vi "SV TDMS Read Position Info.vi"(0 "tdms file":refnum<k34>, 5 "group name in":string, 7 "channel name in":string, 11 "error in":errorcluster) -> (4 "tdms file out":refnum<k34>, 6 "group name out":string, 8 "channel name out":string, 10 "position info":T1, 15 "error out":errorcluster)   [LabVIEW 2017]
uses:
  <vilib>/addons/_NISVFA/_Shared subVIs/Controls/svc_Position Info.ctl
  <vilib>/addons/_NISVFA/_Shared subVIs/Controls/SV Channel Properties.ctl
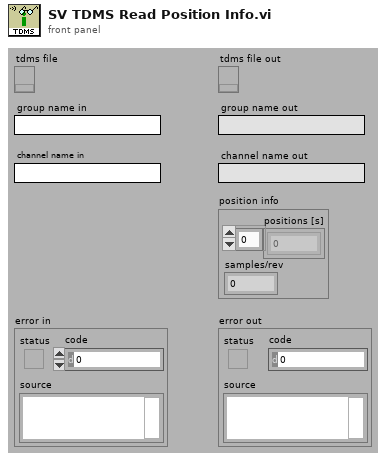
[diagram p1: front panel]
types:
  T1 = typedef "svc_Position Info.ctl" = cluster{"positions [s]":dbl[], "samples/rev":dbl}
  T2 = typedef "SV Channel Properties.ctl" = u16
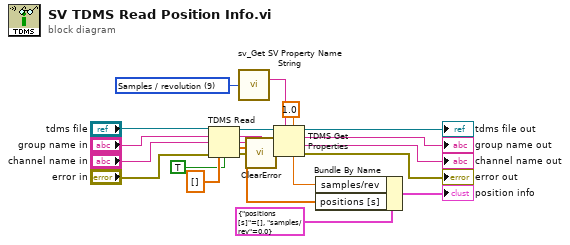
[diagram p0: block diagram]
diagram:
  w16 = T2 9 items=["Engineering units", "Custom unit label", "Weighting filter", "Pregain", "Octave standard", "Octave bandwidth", "Octave low band", "Octave high band", "Spectrum skewed", "Samples / revolution"] ("SV property")
  n1 = TDMS Read(0:"tdms file", 5:"group name in", 7:"channel name in", 11:"error in", 12:dbl[] [] ("positions [s]"), 13:TRUE ("return channels in file order? (F)")) -> (4:w20:refnum<k34>, 6:w22:string, 8:w12:string, 10:w10:dbl[], 15:w2:errorcluster)  [unwired: 2 in, 1 out]
  n2 = call <vilib>:"sv_Get SV Property Name String.vi"("property"=w16) -> ("TDMS property name"=w15:string)  [unwired: 13 in, 1 out]
  n3 = call <vilib>:"ClearError.vi"("error in (no error)"=w2) -> ("error out"=w21:errorcluster)
  n4 = TDMS Get Properties(5:1.0 ("time [s]"), 7:w15, 8:w21, 9:w12, 10:w22, 11:w20) -> (0:→"error out":errorcluster, 1:→"channel name out":string, 2:→"group name out":string, 3:→"tdms file out":refnum<k34>, 4:w3:dbl)  [unwired: 1 out]
  n5 = Bundle By Name(cluster=T1 {"positions [s]"=[], "samples/rev"=0.0} ("speed position info"), "samples/rev"=w3, "positions [s]"=w10) -> (→"position info":T1)
